vi "Draw Bass Clef.vi"(6 "Line Spacing":i16=30, 8 "Start y":i16=430, 9 "Start x":i16=80, 10 "Picture Path":path=path "C:/Users/jag2k2/Desktop/Flashcards", 11 "Picture In":picture) -> (3 "Picture Out":picture)   [LabVIEW 2014]
panel:
  in  "y":i16=-120
  in  "x":i16=15
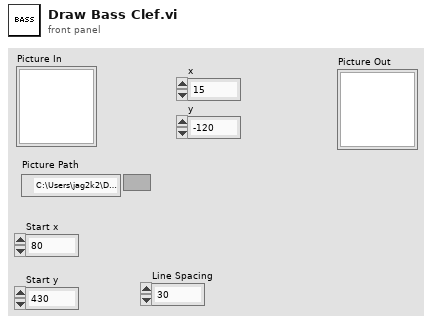
[diagram p1: front panel]
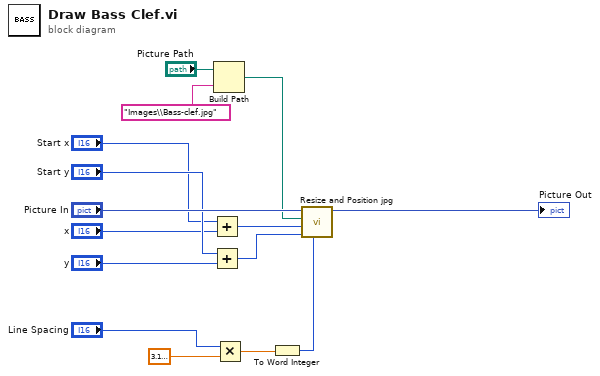
[diagram p0: block diagram]
diagram:
  n1 = Add(x="Start x", y="x") -> (x+y=w8:i16)
  n2 = Add(x="Start y", y="y") -> (x+y=w15:i16)
  n3 = Build Path(base path="Picture Path", name or relative path="Images\\Bass-clef.jpg") -> (appended path=w13:path)
  n4 = Multiply(x="Line Spacing", y=3.1999999999999997 ("y 2")) -> (x*y=w2:dbl)
  n5 = To Word Integer(number=w2) -> (16bit integer=w1:i16)
  n6 = call "Resize and Position jpg.vi"("New Height"=w1, "Pos y"=w15, "Pos x"=w8, "appended path"=w13, "Picture In"="Picture In") -> ("Picture Out"=→"Picture Out":picture)  [unwired: 6 in]
